vi "Configure Qualify Trigger.vi"(0 "VISA resource name":refnum<visa-resource-name>, 1 "Trigger Slope (0: Rising)":u16(ring) items=["Rising", "Falling"], 2 "Trigger Source (0: Channel 1)":u16(ring) items=["Channel 1", "Channel 2", "Channel 3", "Channel 4", "External", "Line", "Ext", "Ext10"], 3 "Trigger Source After Qualifier (1: Channel 2)":u16(ring)=1 items=["Channel 1", "Channel 2", "Channel 3", "Channel 4", "External", "Line", "Ext", "Ext10"], 5 "Trigger Level (0.0 V)":dbl, 7 "Trigger Level 2 (0.0 V)":dbl, 9 "Holdoff Type(0: TI)":u16(ring) items=["TI", "TL", "Events", "None"], 11 "error in (no error)":errorcluster, 12 "Holdoff Value by Time (10 ns)":dbl=1e-08, 14 "Holdoff Value by Events (1)":i32=1) -> (4 "VISA resource name out":refnum<visa-resource-name>, 15 "error out":errorcluster)   [LabVIEW 2015, in "LeCroy Wave Series.lvlib"]
doc: "Configures qualify trigger settings. The Qualify trigger is an edge-qualified SMART Trigger that allows you to use one signal's positive or negative transition to qualify a second signal, which is the trigger source. For Qualify trigger, you specify the time or number of events after the transition when you want the trigger to occur.\n\nNote: \"External\" is included for the purpose of backwards compatibility. Use EXT or EXT10 for best results."
uses:
  <instrlib>/LeCroy Wave Series/LeCroy Wave Series.lvlib
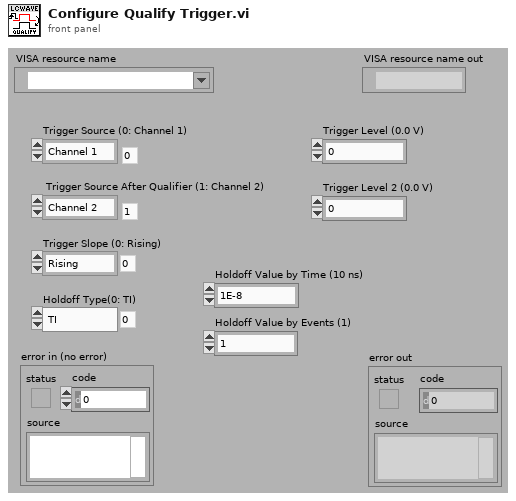
[diagram p1: front panel]
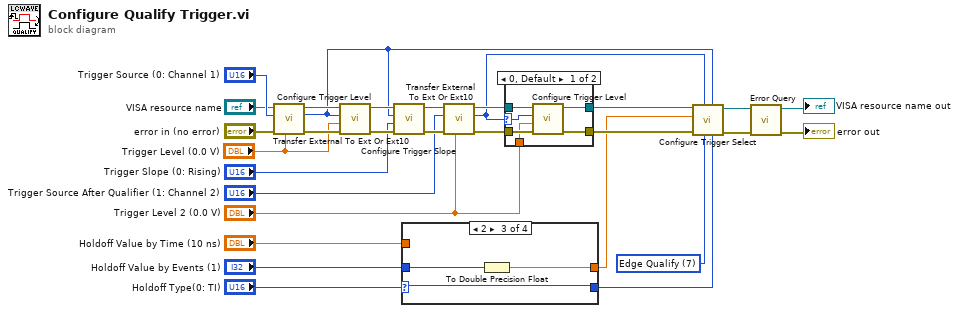
[diagram p0: block diagram]
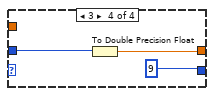
[diagram p5: hidden frame]
diagram:
  w3 = u16 7 items=["Edge", "Dropout", "Glitch", "Interval", "Std", "Sng", "State Qualify", "Edge Qualify"] ("Trigger type")
  n1 = call <instrlib>:"Transfer External To Ext Or Ext10.vi"("Trigger Level"="Trigger Level (0.0 V)", "error in (no error)"="error in (no error)", "Trigger Source With External"="Trigger Source (0: Channel 1)", "VISA resource name"="VISA resource name") -> ("error out"=w16:errorcluster, "Trigger Source With Ext/Ext10"=w1:u16, "VISA resource name out"=w15:refnum<visa-resource-name>)  [unwired: 5 in]
  n2 = call <instrlib>:"Configure Trigger Level.vi"("error in (no error)"=w16, "Trigger Level 1 (0.0 V)"="Trigger Level (0.0 V)", "Channel (0: Channel 1)"=w1, "VISA resource name"=w15) -> ("error out"=w28:errorcluster, "VISA resource name out"=w29:refnum<visa-resource-name>)  [unwired: 6 in]
  n3 = call <instrlib>:"Configure Trigger Slope.vi"("error in (no error)"=w28, "Trigger Slope (0: Rising)"="Trigger Slope (0: Rising)", "Channel (0: Channel 1)"=w1, "VISA resource name"=w29) -> ("error out"=w9:errorcluster, "VISA resource name out"=w11:refnum<visa-resource-name>)  [unwired: 6 in]
  n4 = case shown="2" "Holdoff Type(0: TI)" {
    selector: "Holdoff Type(0: TI)" -> [w30 w32 w36 _]
    tunnel: "Holdoff Value by Time (10 ns)" -> [w31 w33 _ _]
    tunnel: "Holdoff Value by Events (1)" -> [_ _ w35 w38]
    tunnel: [w31 w33 w34 w37] -> w21
    tunnel: [w30 w32 w36 9] -> w4
    frame 0, Default {
    }
    frame 1 {
    }
    frame 2 {
      n5 = To Double Precision Float(number=w35) -> (double precision float=w34:dbl)
    }
    frame 3 {
      n6 = To Double Precision Float(number=w38) -> (double precision float=w37:dbl)
    }
  }
  n7 = call <instrlib>:"Transfer External To Ext Or Ext10.vi"("Trigger Level"="Trigger Level 2 (0.0 V)", "error in (no error)"=w9, "Trigger Source With External"="Trigger Source After Qualifier (1: Channel 2)", "VISA resource name"=w11) -> ("error out"=w8:errorcluster, "Trigger Source With Ext/Ext10"=w2:u16, "VISA resource name out"=w10:refnum<visa-resource-name>)  [unwired: 5 in]
  n8 = case shown="0, Default" w2 {
    selector: w2 -> [w40 _]
    tunnel: w10 -> [w45 w47]
    tunnel: w8 -> [w44 w46]
    tunnel: [w43 w47] -> w26
    tunnel: [w42 w46] -> w25
    tunnel: "Trigger Level 2 (0.0 V)" -> [w41 _]
    frame 0, Default {
      n9 = call <instrlib>:"Configure Trigger Level.vi"("error in (no error)"=w44, "Trigger Level 1 (0.0 V)"=w41, "Channel (0: Channel 1)"=w40, "VISA resource name"=w45) -> ("error out"=w42:errorcluster, "VISA resource name out"=w43:refnum<visa-resource-name>)  [unwired: 6 in]
    }
    frame 6 {
    }
  }
  n10 = call <instrlib>:"Configure Trigger Select.vi"("Hold Type (0: TI)"=w4, "QL (1: Channel 2)"=w1, "Trigger type"=w3, "Trigger Source (0: Channel 1)"=w2, "error in (no error)"=w25, "Hold Value 1 (4 ns)"=w21, "VISA resource name"=w26) -> ("error out"=w17:errorcluster, "VISA resource name out"=w18:refnum<visa-resource-name>)  [unwired: 3 in]
  n11 = call <instrlib>:"Error Query.vi"("error in (no error)"=w17, "VISA resource name"=w18) -> ("error out"=→"error out":errorcluster, "VISA resource name out"=→"VISA resource name out":refnum<visa-resource-name>)  [unwired: 6 in, 2 out]
